vi "apply mapping changes.vi"(4 "original channel":refnum<class "TBM channel.lvclass">, 6 "original tag":refnum<class "tag descriptor.lvclass">, 7 "owner ID":string, 8 "error in":errorcluster, 9 "channel":refnum<class "TBM channel.lvclass">, 10 "tag descriptor":refnum<class "tag descriptor.lvclass">, 11 "engine configuration in":refnum<class "Simple Sequencer TBM configuration.lvclass">) -> (0 "error out":errorcluster, 3 "engine configuration out":refnum<class "Simple Sequencer TBM configuration.lvclass">)   [LabVIEW 2014, in "Simple Sequencer TBM configuration.lvclass"]
uses:
  <vilib>/NI/TBM Modules/Sequencer/module/configuration/Simple Sequencer TBM configuration.lvclass
  <vilib>/NI/Tag Bus/tag/tag descriptor.lvclass
  <vilib>/NI/Tag Bus Module Framework/channel/TBM channel.lvclass
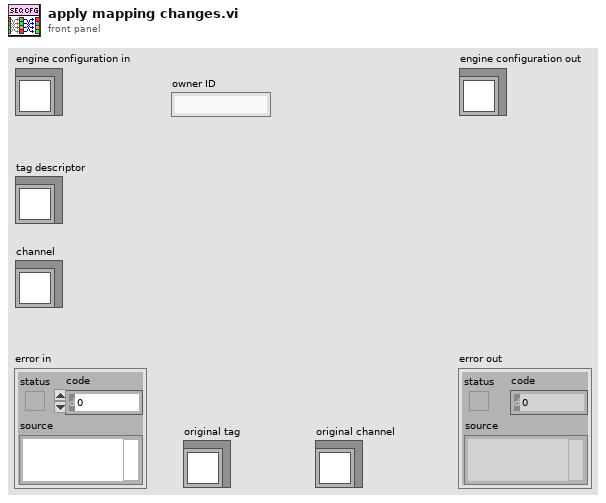
[diagram p1: front panel]
types:
  T1 = typedef "TBM channel.lvclass/channel classification.ctl" = enum16{"input data", "output data", "processing parameter", "processing result"}
  T2 = typedef "tag bus.lvlib/tag descriptor.lvclass/Data Type.ctl" = enum16{"Double", "Single", "I64", "I32", "I16", "I8", "U64", "U32", "U16", "U8", "Boolean", "String", "Array of Double", "Array of Single", "Array of I64", "Array of I32", "Array of I16", "Array of I8", "Array of U64", "Array of U32", "Array of U16", "Array of U8", "Array of Boolean", "Array of String"}
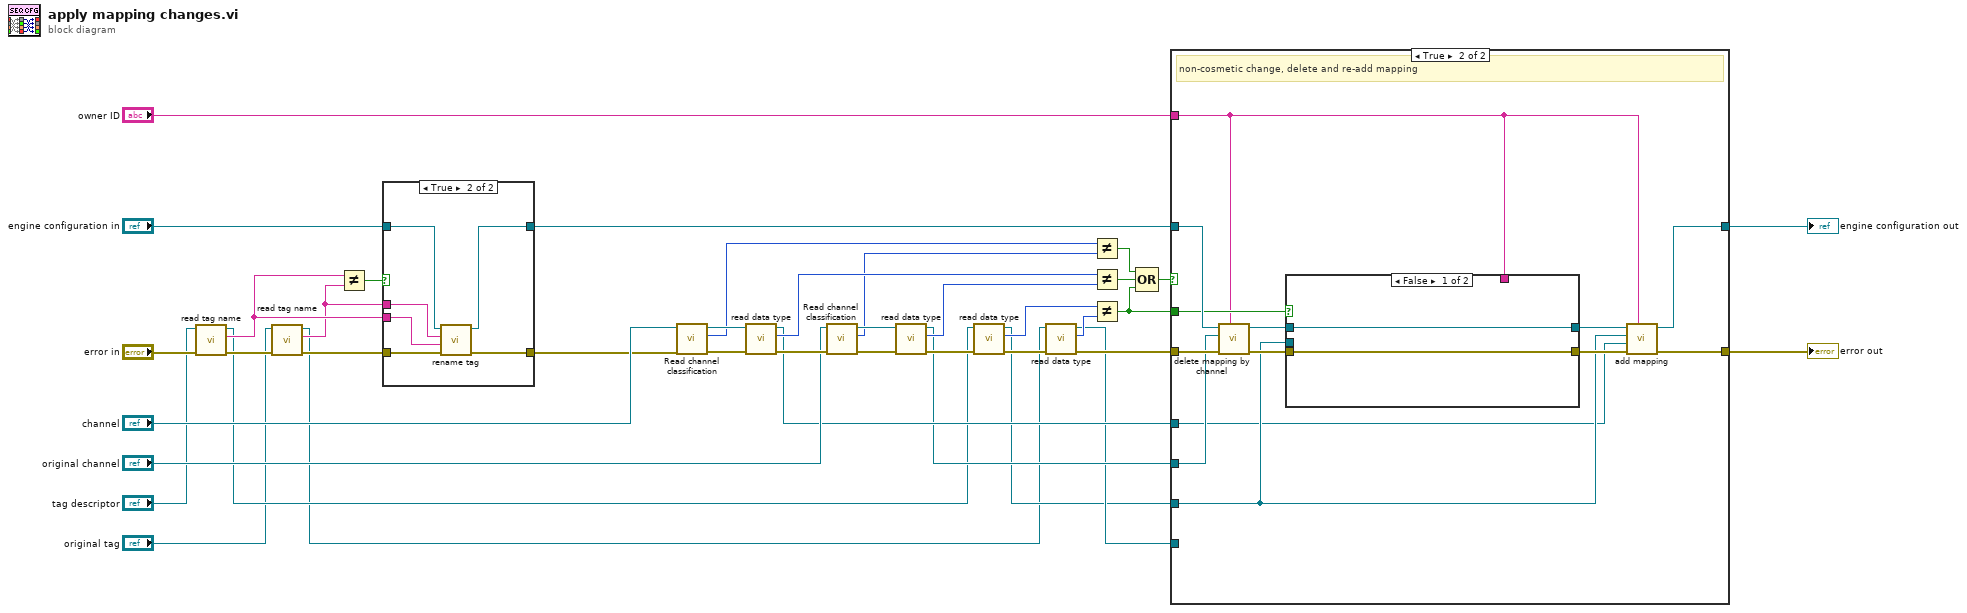
[diagram p0: block diagram]
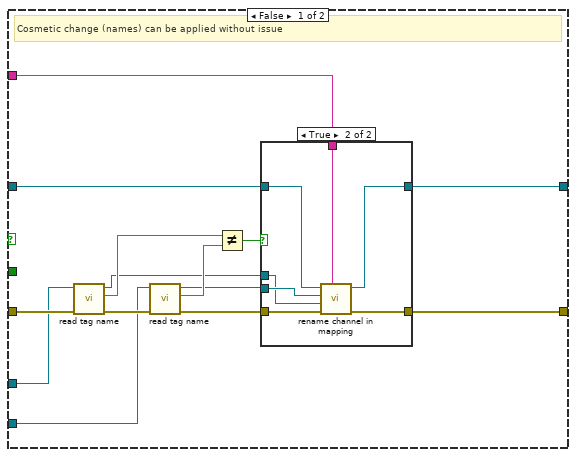
[diagram p3: hidden frame]
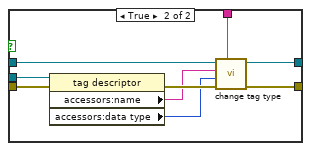
[diagram p5: hidden frame]
diagram:
  n1 = call <vilib>:"read tag name.vi"("error in"="error in", "system tag in"="tag descriptor") -> ("error out"=w11:errorcluster, "name"=w13:string, "system tag out"=w3:refnum<class "tag descriptor.lvclass">)  [unwired: 7 in]
  n2 = call <vilib>:"read tag name.vi"("error in"=w11, "system tag in"="original tag") -> ("error out"=w10:errorcluster, "name"=w12:string, "system tag out"=w1:refnum<class "tag descriptor.lvclass">)  [unwired: 7 in]
  n3 = Not Equal?(x=w13, y=w12) -> (x != y?=w9:bool)
  n4 = case shown="True" w9 {
    tunnel: w10 -> [w42 w46]
    tunnel: [w41 w44] -> w6
    tunnel: [w42 w45] -> w5
    tunnel: w12 -> [_ w47]
    tunnel: w13 -> [_ w48]
    tunnel: "engine configuration in" -> [w41 w43]
    frame False {
    }
    frame True {
      n5 = call <vilib>:"rename tag.vi"("error in"=w46, "new name"=w48, "old name"=w47, "engine configuration in"=w43) -> ("error out"=w45:errorcluster, "engine configuration out"=w44:refnum<class "Simple Sequencer TBM configuration.lvclass">)  [unwired: 6 in]
    }
  }
  n6 = call <vilib>:"Read channel classification.vi"("error in"=w5, "channel in"="channel") -> ("error out"=w38:errorcluster, "channel classification"=w24:T1, "channel out"=w39:refnum<class "TBM channel.lvclass">)  [unwired: 7 in]
  n7 = call <vilib>:"read data type.vi"("error in"=w38, "system tag in"=w39) -> ("error out"=w35:errorcluster, "data type"=w26:T2, "system tag out"=w21:refnum<class "TBM channel.lvclass">)  [unwired: 7 in]
  n8 = call <vilib>:"Read channel classification.vi"("error in"=w35, "channel in"="original channel") -> ("error out"=w37:errorcluster, "channel classification"=w25:T1, "channel out"=w36:refnum<class "TBM channel.lvclass">)  [unwired: 7 in]
  n9 = call <vilib>:"read data type.vi"("error in"=w37, "system tag in"=w36) -> ("error out"=w33:errorcluster, "data type"=w27:T2, "system tag out"=w20:refnum<class "TBM channel.lvclass">)  [unwired: 7 in]
  n10 = call <vilib>:"read data type.vi"("error in"=w33, "system tag in"=w3) -> ("error out"=w32:errorcluster, "data type"=w28:T2, "system tag out"=w18:refnum<class "tag descriptor.lvclass">)  [unwired: 7 in]
  n11 = call <vilib>:"read data type.vi"("error in"=w32, "system tag in"=w1) -> ("error out"=w22:errorcluster, "data type"=w29:T2, "system tag out"=w19:refnum<class "tag descriptor.lvclass">)  [unwired: 7 in]
  n12 = Not Equal?(x=w24, y=w25) -> (x != y?=w30:bool)
  n13 = Not Equal?(x=w26, y=w27) -> (x != y?=w31:bool)
  n14 = Not Equal?(x=w28, y=w29) -> (x != y?=w17:bool)
  n15 = Compound Arithmetic op=OR(w30, w31, w17) -> (w23:bool)
  n16 = case shown="True" w23 {
    tunnel: w22 -> [w53 w84]
    tunnel: w21 -> [w50 w72]
    tunnel: w20 -> [w49 w82]
    tunnel: w19 -> [_ _]
    tunnel: w18 -> [_ w73]
    tunnel: w17 -> [_ w81]
    tunnel: w6 -> [w51 w83]
    tunnel: [w55 w76] -> w16
    tunnel: [w54 w75] -> w15
    tunnel: "owner ID" -> [w52 w74]
    frame False {
      # "Cosmetic change (names) can be applied without issue"
      n17 = call <vilib>:"read tag name.vi"("error in"=w53, "system tag in"=w50) -> ("error out"=w62:errorcluster, "name"=w60:string, "system tag out"=w56:refnum<class "TBM channel.lvclass">)  [unwired: 7 in]
      n18 = call <vilib>:"read tag name.vi"("error in"=w62, "system tag in"=w49) -> ("error out"=w59:errorcluster, "name"=w61:string, "system tag out"=w57:refnum<class "TBM channel.lvclass">)  [unwired: 7 in]
      n19 = Not Equal?(x=w60, y=w61) -> (x != y?=w58:bool)
      n20 = case shown="True" w58 {
        tunnel: w59 -> [w63 w71]
        tunnel: w51 -> [w64 w70]
        tunnel: w52 -> [_ w69]
        tunnel: w57 -> [_ w68]
        tunnel: w56 -> [_ w67]
        tunnel: [w64 w66] -> w54
        tunnel: [w63 w65] -> w55
        frame False {
        }
        frame True {
          n21 = call <vilib>:"rename channel in mapping.vi"("owner ID"=w69, "error in"=w71, "new action channel"=w67, "old action channel"=w68, "engine configuration in"=w70) -> ("error out"=w65:errorcluster, "engine configuration out"=w66:refnum<class "Simple Sequencer TBM configuration.lvclass">)  [unwired: 5 in]
        }
      }
    }
    frame True {
      # "non-cosmetic change, delete and re-add mapping"
      n22 = call <vilib>:"delete mapping by channel.vi"("owner ID"=w74, "error in"=w84, "action channel"=w82, "engine configuration in"=w83) -> ("error out"=w79:errorcluster, "engine configuration out"=w80:refnum<class "Simple Sequencer TBM configuration.lvclass">)  [unwired: 6 in]
      n23 = case shown="False" w81 {
        tunnel: w80 -> [w86 w95]
        tunnel: w74 -> [_ w94]
        tunnel: w79 -> [w85 w93]
        tunnel: w73 -> [_ w91]
        tunnel: [w85 w88] -> w77
        tunnel: [w86 w87] -> w78
        frame False {
        }
        frame True {
          n24 = property class="tag descriptor"(reference=w91, error in=w93) -> (error out=w92:errorcluster, "accessors:name"=w89:string, "accessors:data type"=w90:T2)  [unwired: 1 out]
          n25 = call <vilib>:"change tag type.vi"("owner ID"=w94, "error in"=w92, "new data type"=w90, "tag name"=w89, "engine configuration in"=w95) -> ("error out"=w88:errorcluster, "engine configuration out"=w87:refnum<class "Simple Sequencer TBM configuration.lvclass">)  [unwired: 5 in]
        }
      }
      n26 = call <vilib>:"add mapping.vi"("owner ID"=w74, "error in"=w77, "action channel"=w72, "channel descriptor"=w73, "engine configuration"=w78) -> ("error out"=w76:errorcluster, "engine configuration out"=w75:refnum<class "Simple Sequencer TBM configuration.lvclass">)  [unwired: 5 in]
    }
  }
  "error out" <- w16
  "engine configuration out" <- w15
